vi "Slice String__ogtk.vi"(2 "include string[j]":bool caption="include string[j] (false)", 5 "slice":string caption="subset (i:j)", 6 "string":string) -> (1 "substring":string caption="substring (string[i:j])")   [LabVIEW 2009]
doc: "<b>This VI Is Depreciated</b> \nPlease use \"Slice String 1.vi\" (or newer version), available as \"Slice String\" from the Functions Palette.\n\n\nReturns a <B>substring</B>, specified by <B>subset</B>, from <B>string</B>. \n\nSlice String.vi was originally written to emulate the slice notation of Python. (See below for extended capabilities.) In Python, a slice is a subset of elements in a list and a string is a list of characters. If you want to access one character in the string (or one element in any list), you'd use the list name and the index value:\n\n<B>substring</B> = <B>string</B>[i]\n\nTo get multple contiguous characters, use the slice i:j notation in place of the single index:\n\n<B>substring</B> = <B>string</B>[i:j]\n\nCharacters (elements) are assigned to the output starting at the first index value, and continuing up to, but not including, the last value.\n\nIn this notation, i and j are integers.\nThe first character in <B>string</B> has index zero.\nIf i is ommitted it is assumed to be zero and <B>substring</B>contains the leftmost characters of <B>string</B>.\nIf j is ommitted it is assumed to be length(string) and <B>substring</B>contains the rightmost characters of <B>string</B>.\nIf i or j are negative numbers they are assumed to be referenced from the end of the string.\n\nIn the LabVIEW implementation, the range of the slice is expressed in the string variable <B>subset</B> as \"i:j\".\n\nSlice String.vi has now been extended to allow the (optional) inclusion of the last value as well (for those who are used to the closed interval syntax) by wiring a TRUE constant to the fourth terminal. (Only two of the examples below, in boldface, are affected.)\n\nExamples:\n\nIf <B>string</B> = \"MyString\" \nfor <B>include string[j]</B> = FALSE (default) / for <B>include string[j]</B> = TRUE\n\nstring[2:] = \"String\" string[2:] = \"String\"\nstring[:3] = \"MyS\" string[:3] = \"<B>MySt</B>\"\nstring[-1] = \"g\" string[-1] = \"g\"\nstring[4] = \"r\" string[4] = \"r\"\nstring[-4:-2] = \"ri\" string[-4:-2] = \"<B>rin</B>\""
panel:
  # "Please visit http://www.OpenG.org to learn about the\nOpen Source LabVIEW software movement.\n\nNOTICE -- YOU MUST LEAVE THIS NOTICE IN PLACE.  PER THE TERMS OF THE LICENSE BELOW, YOU MAY SUBLICENSE THIS SOFTWARE \nIN ANY WAY THAT DOES NOT CONFLICT WITH THIS LICENSE.\n\n### BSD License (http://www.opensource.org/licenses/bsd-license.php) Begin ###\n \nCopyright (c) 2002, Jim Kring <jim@jimkring.com>\nCopyright (c) 2002, Cal-Bay Systems, Inc. <info@calbay.com>\nCopyright (c) 2004, Paul F. Sullivan <Paul@SULLutions.com>\nCopyright (c) 2011, Jonathon Green <jg@jgcode.net>\n\nAll rights reserved.\n\nRedistribution and use in source and binary forms, with or without modification, are permitted provided that the following conditions are met:\n\n    * Redistributions of source code must retain the above copyright notice, this list of conditions and the following disclaimer.\n    * Redistributions in binary form must reproduce the above copyright notice, this list of conditions and the following disclaimer in the \n       documentation and/or other materials provided with the distribution.\n    * Neither the name of SciWare, James Kring, Inc., nor the names of its contributors may be used to endorse or promote products derived \n       from this software without specific prior written permission.\n\nTHIS SOFTWARE IS PROVIDED BY THE COPYRIGHT HOLDERS AND CONTRIBUTORS \"AS IS\" AND ANY EXPRESS OR IMPLIED WARRANTIES, \nINCLUDING, BUT NOT LIMITED TO, THE IMPLIED WARRANTIES OF MERCHANTABILITY AND FITNESS FOR A PARTICULAR PURPOSE ARE \nDISCLAIMED. IN NO EVENT SHALL THE COPYRIGHT OWNER OR CONTRIBUTORS BE LIABLE FOR ANY DIRECT, INDIRECT, INCIDENTAL,\n SPECIAL, EXEMPLARY, OR CONSEQUENTIAL DAMAGES (INCLUDING, BUT NOT LIMITED TO, PROCUREMENT OF SUBSTITUTE GOODS OR \nSERVICES; LOSS OF USE, DATA, OR PROFITS; OR BUSINESS INTERRUPTION) HOWEVER CAUSED AND ON ANY THEORY OF LIABILITY, \nWHETHER IN CONTRACT, STRICT LIABILITY, OR TORT (INCLUDING NEGLIGENCE OR OTHERWISE) ARISING IN ANY WAY OUT OF THE USE \nOF THIS SOFTWARE, EVEN IF ADVISED OF THE POSSIBILITY OF SUCH DAMAGE.\n\n### BSD License End ###"
  # "This VI Is Depreciated. \nPlease use \"Slice String 1.vi\" (or newer version), available as \"Slice String\" from the Functions Palette."
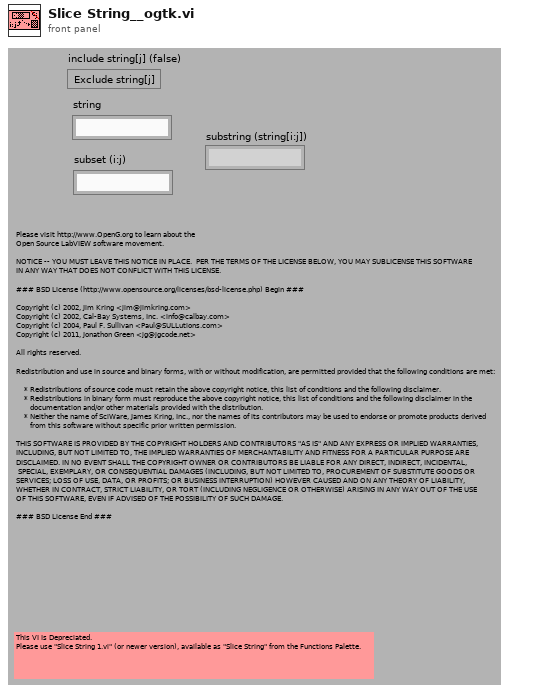
[diagram p1: front panel]
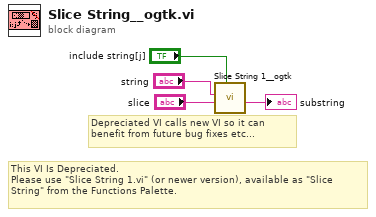
[diagram p0: block diagram]
diagram:
  # "Depreciated VI calls new VI so it can benefit from future bug fixes etc..."
  # "This VI Is Depreciated. \nPlease use \"Slice String 1.vi\" (or newer version), available as \"Slice String\" from the Functions Palette."
  n1 = call "Slice String 1__ogtk.vi"("Include String[j] (false)"="include string[j]", "Subset (i:j)"="slice", "String"="string") -> ("Substring (String[i:j])"=→"substring":string)  [unwired: 6 in]
